vi "Write Bias Voltage (V).vi"(10 "Bias Voltage (V)":dbl, 11 "LCR Meter in":refnum<class "LCR Meter.lvclass">) -> (3 "LCR Meter out":refnum<class "LCR Meter.lvclass">)   [LabVIEW 2020, in "LCR Meter.lvclass"]
uses:
  LCR Meter.lvclass
  LCR Meter.lvclass/LCR Meter.ctl
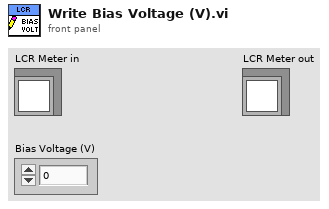
[diagram p1: front panel]
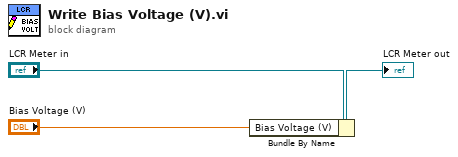
[diagram p0: block diagram]
diagram:
  n1 = Bundle By Name(cluster="LCR Meter in", "Bias Voltage (V)"="Bias Voltage (V)") -> (→"LCR Meter out":refnum<class "LCR Meter.lvclass">)
